vi "Get Glyph Slot Ref.vi"(8 "error in (no error)":errorcluster, 11 "face in":i64) -> (0 "error out":errorcluster, 2 "glyph slot ref":i64, 3 "face out":i64)   [LabVIEW 2023, in "Freetype Drawer.lvlib"]
uses:
  Freetype Drawer.lvlib
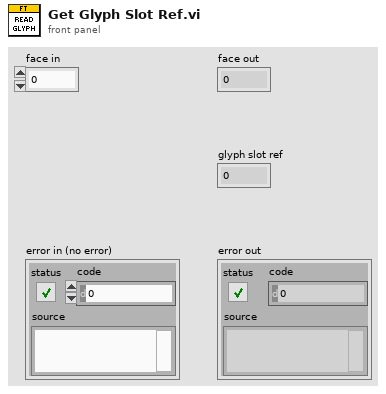
[diagram p1: front panel]
types:
  T1 = typedef "Freetype Drawer.lvlib/Face.ctl" = cluster{"num_faces":i32, "face_index":i32, "face_flags":i32, "style_flags":i32, "num_glyphs":i32, "family_name":i64, "style_name":i64, "num_fixed_sizes":i32, "available_sizes":i64, "num_charmaps":i32, "charmaps":i64, "generic":cluster{"pointer":i64, "finalizer":i64}, "bbox":cluster{"xmin":i32, "ymin":i32, "xmax":i32, "ymax":i32}, "units_per_em":u16, "ascender":i16, "descender":i16, "height":i16, "max_advance_width":i16, "max_advance_height":i16, "underline_position":i16, "underline_thickness":i16, "glyph":i64, "size":i64, "charmap":i64}
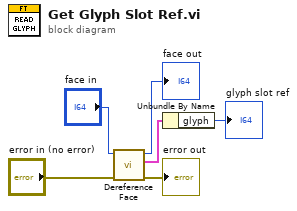
[diagram p0: block diagram]
diagram:
  n1 = call "Dereference Face.vi"("error in (no error)"="error in (no error)", "face in"="face in") -> ("error out"=→"error out":errorcluster, "Face"=w5:T1, "face out"=→"face out":i64)  [unwired: 7 in]
  n2 = Unbundle By Name(w5) -> ("glyph"=→"glyph slot ref":i64)
